vi "Xcorimages (SubVI).vi"(5 "error out":errorcluster, 7 "ROI smooth template in":dbl[][](array[numeric]), 8 "Bead template in":dbl[][](array[numeric]), 10 "multi image in":i32[][](array[numeric])) -> (0 "error out 2":errorcluster, 2 "Array":dbl[][](array[numeric]))   [LabVIEW 2011]
uses:
  <vilib>/Analysis/2dsp.llb/2D Real FFT.vi
  <vilib>/Analysis/2dsp.llb/2D Inverse Real FFT.vi
  <vilib>/Analysis/NI_AALPro.lvlib
  <vilib>/Analysis/NI_AALBase.lvlib
panel:
  out "ori image 6":i32[][](graph)
  out "ori image 5":dbl[][](graph)
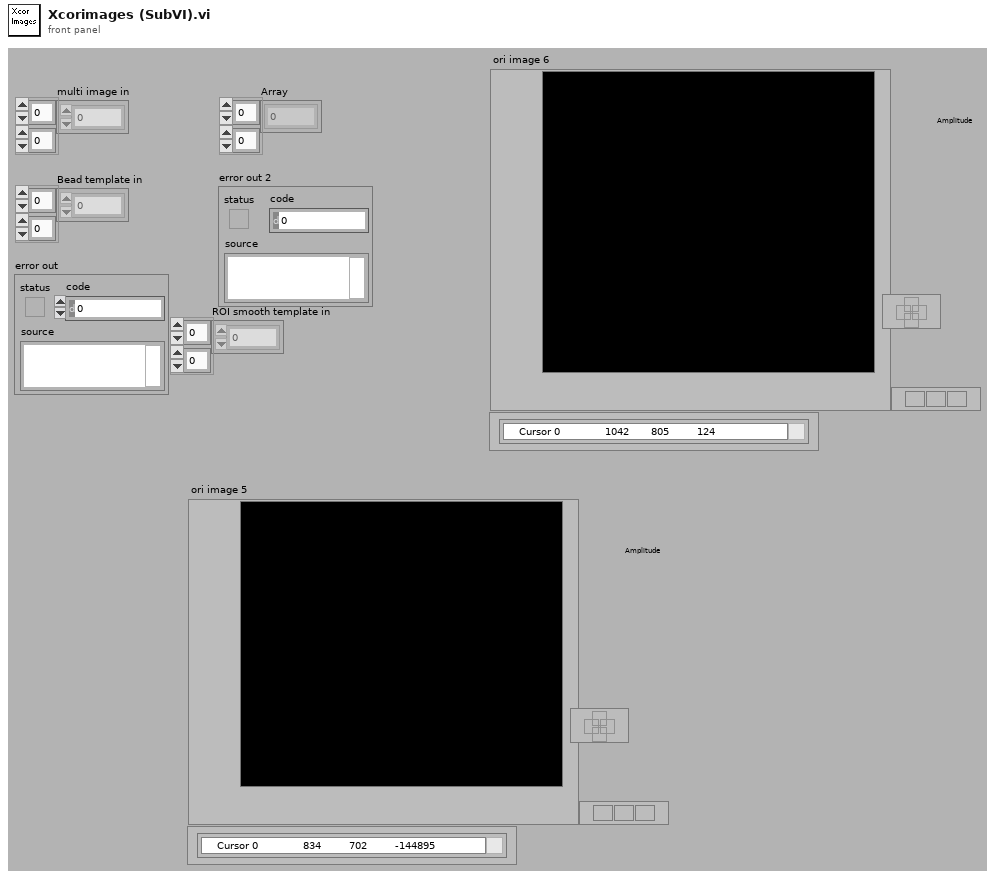
[diagram p1: front panel]
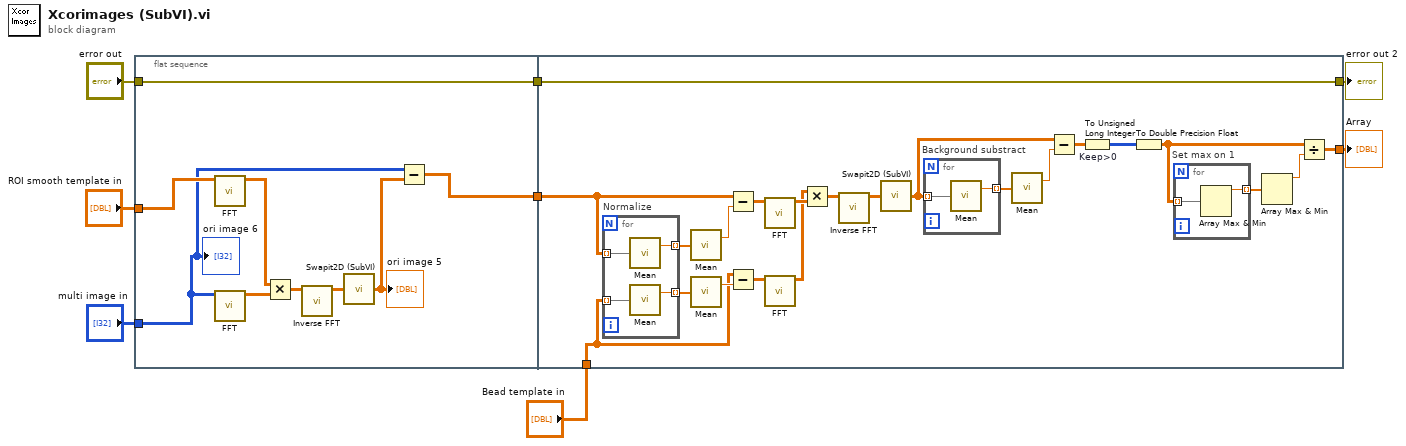
[diagram p0: block diagram]
diagram:
  n1 = flat-sequence {
    tunnel: "multi image in" -> [w9]
    tunnel: "ROI smooth template in" -> [w10]
    tunnel: [w11] -> w6
    tunnel: "error out" -> [w13]
    tunnel: [w13] -> w2
    tunnel: [w19] -> w7
    tunnel: w6 -> [w20]
    tunnel: "Bead template in" -> [w21]
    tunnel: [w18] -> w1
    tunnel: w2 -> [w18]
    frame #0 {
      n2 = call-poly <vilib>:"FFT.vi"("X"=w10) -> ("FFT {X}"=w14:cdb[][])  [unwired: 3 in, 7 out]
      n3 = call-poly <vilib>:"FFT.vi"("X"=w9) -> ("FFT {X}"=w15:cdb[][])  [unwired: 3 in, 7 out]
      n4 = Multiply(x=w14, y=w15) -> (x*y=w16:cdb[][])
      n5 = call-poly <vilib>:"Inverse FFT.vi"("FFT {X}"=w16) -> ("X"=w17:dbl[][])  [unwired: 1 in, 9 out]
      n6 = call "Swapit2D (SubVI).vi"("oriplot"=w17) -> ("Zero-centerd Xcor"=w12:dbl[][])
      "ori image 5" <- w12
      n7 = Subtract(x=w9, y=w12) -> (x-y=w11:dbl[][])
      "ori image 6" <- w9
    }
    frame #1 {
      n8 = for "Normalize" {
        tunnel: w21 -> [w47] mode=indexing
        tunnel: [w46] -> w26 mode=indexing
        tunnel: w20 -> [w45] mode=indexing
        tunnel: [w44] -> w29 mode=indexing
        n9 = call <vilib>:"Mean.vi"("X"=w45) -> ("mean"=w44:dbl)  [unwired: 1 out]
        n10 = call <vilib>:"Mean.vi"("X"=w47) -> ("mean"=w46:dbl)  [unwired: 1 out]
      }
      n11 = call <vilib>:"Mean.vi"("X"=w29) -> ("mean"=w28:dbl)  [unwired: 1 out]
      n12 = call <vilib>:"Mean.vi"("X"=w26) -> ("mean"=w27:dbl)  [unwired: 1 out]
      n13 = Subtract(x=w20, y=w28) -> (x-y=w31:dbl[][])
      n14 = Subtract(x=w21, y=w27) -> (x-y=w30:dbl[][])
      n15 = call-poly <vilib>:"FFT.vi"("X"=w31) -> ("FFT {X}"=w23:cdb[][])  [unwired: 3 in, 7 out]
      n16 = call-poly <vilib>:"FFT.vi"("X"=w30) -> ("FFT {X}"=w22:cdb[][])  [unwired: 3 in, 7 out]
      n17 = Multiply(x=w22, y=w23) -> (x*y=w24:cdb[][])
      n18 = call-poly <vilib>:"Inverse FFT.vi"("FFT {X}"=w24) -> ("X"=w25:dbl[][])  [unwired: 1 in, 9 out]
      n19 = call "Swapit2D (SubVI).vi"("oriplot"=w25) -> ("Zero-centerd Xcor"=w32:dbl[][])
      n20 = for "Background substract" {
        tunnel: w32 -> [w43] mode=indexing
        tunnel: [w42] -> w35 mode=indexing
        n21 = call <vilib>:"Mean.vi"("X"=w43) -> ("mean"=w42:dbl)  [unwired: 1 out]
      }
      n22 = call <vilib>:"Mean.vi"("X"=w35) -> ("mean"=w36:dbl)  [unwired: 1 out]
      n23 = Subtract(x=w32, y=w36) -> (x-y=w38:dbl[][])
      n24 = To Unsigned Long Integer "Keep>0"(number=w38) -> (unsigned 32bit integer=w37:u32[][])
      n25 = To Double Precision Float(number=w37) -> (double precision float=w39:dbl[][])
      n26 = for "Set max on 1" {
        tunnel: w39 -> [w41] mode=indexing
        tunnel: [w40] -> w33 mode=indexing
        n27 = Array Max & Min(array=w41) -> (max value=w40:dbl)  [unwired: 3 out]
      }
      n28 = Array Max & Min(array=w33) -> (max value=w34:dbl)  [unwired: 3 out]
      n29 = Divide(x=w39, y=w34) -> (x/y=w19:dbl[][])
    }
  }
  "error out 2" <- w1
  "Array" <- w7
